vi "Move.vi"(8 "error in (no error)":errorcluster, 9 "Direction Offset":i32, 10 "Current Position":T3, 11 "Test in":refnum<class "Swarm.lvclass">) -> (0 "error out":errorcluster, 1 "Direction":T1, 2 "Action":T2, 3 "Test out":refnum<class "Swarm.lvclass">)   [LabVIEW 2017, in "Swarm.lvclass"]
uses:
  Swarm.lvclass
  Common/Position.ctl
  Type Defs/Action Enum.ctl
  Type Defs/Direction Enum.ctl
  Swarm.lvclass/Swarm.ctl
  Type Defs/SB Type Defs.lvlib
  Common/Common.lvlib
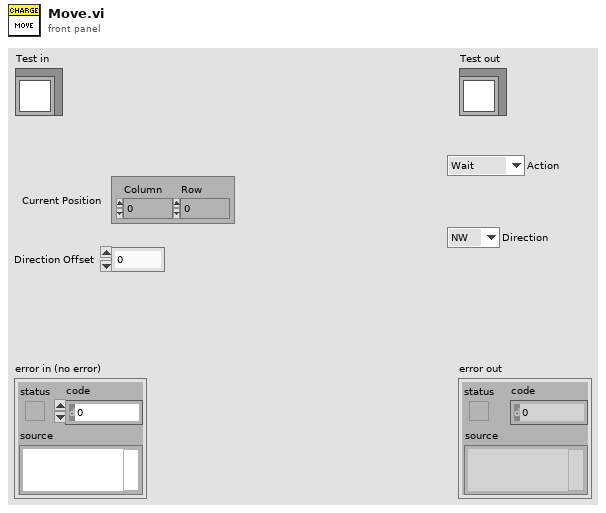
[diagram p1: front panel]
types:
  T1 = typedef "SB Type Defs.lvlib/Direction Enum.ctl" = enum16{"NW", "N", "NE", "E", "SE", "S", "SW", "W"}
  T2 = typedef "SB Type Defs.lvlib/Action Enum.ctl" = enum16{"Wait", "Move", "Attack", "Replicate"}
  T3 = typedef "Common.lvlib/Position.ctl" = cluster{"Column":i32, "Row":i32}
  T4 = typedef "Common.lvlib/Map DVR.ctl" = refnum<data-value>
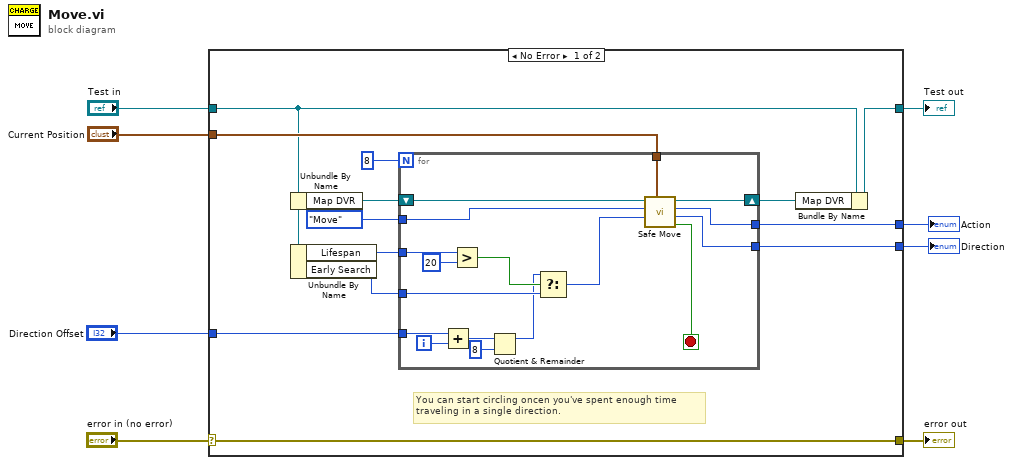
[diagram p0: block diagram]
diagram:
  n1 = case shown="No Error" "error in (no error)" {
    selector: "error in (no error)" -> [w21 w40]
    tunnel: [w21 w40] -> w7
    tunnel: [w16 w39] -> w5
    tunnel: "Test in" -> [w11 w39]
    tunnel: "Direction Offset" -> [w15 _]
    tunnel: "Current Position" -> [w14 _]
    tunnel: [w13 _] -> w2
    tunnel: [w12 _] -> w1
    frame No Error {
      # "You can start circling oncen you've spent enough time\ntraveling in a single direction."
      n2 = Unbundle By Name(w11) -> ("Map DVR"=w19:T4)
      n3 = Unbundle By Name(w11) -> ("Lifespan"=w10:i32, "Early Search"=w9:T1)
      n4 = for {
        N: 8 -> [_]
        tunnel: Action_Enum."Move" ("Desired Action") -> [w38]
        tunnel: w14 -> [w35]
        shift-right: [w36] -> w18
        shift-left: w19 -> [w37]
        tunnel: [w33] -> w13
        tunnel: [w32] -> w12
        tunnel: w15 -> [w28]
        tunnel: w10 -> [w27]
        tunnel: w9 -> [w24]
        i -> [w31]
        stop <- w34 stop-if-true
        n5 = Add(x=w28, y=w31) -> (x+y=w30:i32)
        n6 = Greater?(x=w27, y=20 ("x")) -> (0:w25:bool)
        n7 = Quotient & Remainder(x=w30, y=8) -> (x-y*floor(x/y)=w23:i32)  [unwired: 1 out]
        n8 = Select(t=w23, s=w25, f=w24) -> (s? t:f=w22:i32)
        n9 = call "Safe Move.vi"("Position in"=w35, "Direction in"=w22, "Desired Action"=w38, "Map DVR"=w37) -> ("Accepted?"=w34:bool, "Direction"=w32:T1, "Action"=w33:T2, "Map DVR out"=w36:T4)  [unwired: 4 in]
      }
      n10 = Bundle By Name(cluster=w11, "Map DVR"=w18) -> (w16:refnum<class "Swarm.lvclass">)
    }
    frame Error {
    }
  }
  "error out" <- w7
  "Test out" <- w5
  "Action" <- w2
  "Direction" <- w1
